vi "Thorlabs FWxC Read & Write demo.vi"() -> ()   [LabVIEW 2013]
doc: "This example shows how to acquire a power measurement using the VIs of the driver."
uses:
  <instrlib>/Thorlabs_FWxC/Thorlabs_FWxC.lvlib
panel:
  in  "Set Sensor Mode":T1(ring)
  in  "Set Speed Mode":enum16{"Slow Speed", "High Speed"}(ring)
  in  "Set Trigger Mode":enum16{"Input Mode", "Output Mode"}(ring)
  out "Get Sensor Mode":T1(ring)
  out "COM Ports":string[](array[string])
  out "Get Position":i32
  in  "Set Position":i32=5
  out "Get Speed Mode":enum16{"Slow Speed", "High Speed"}(ring)
  out "Get Trigger Mode":enum16{"Input Mode", "Output Mode"}(ring)
  out "Get Position Count":i32
  out "ID":string
  # "(c) 2020 <Thorlabs>.  ALL RIGHTS RESERVED."
  # "Connect"
  # "Set data"
  # "Read data"
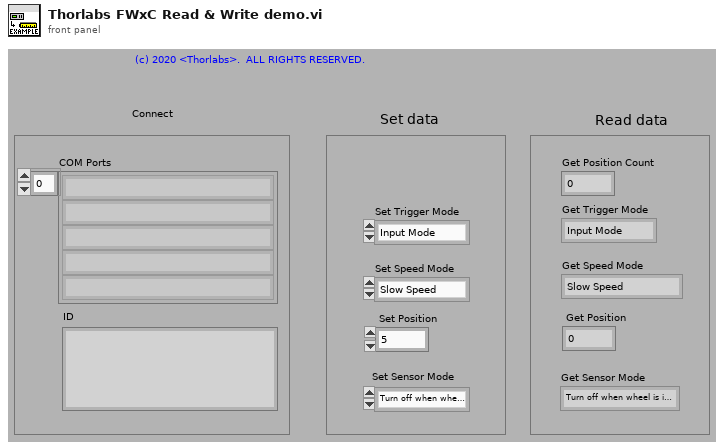
[diagram p1: front panel]
types:
  T1 = enum16{"Turn off when wheel is idle to eliminate stray light", "Remain active"}
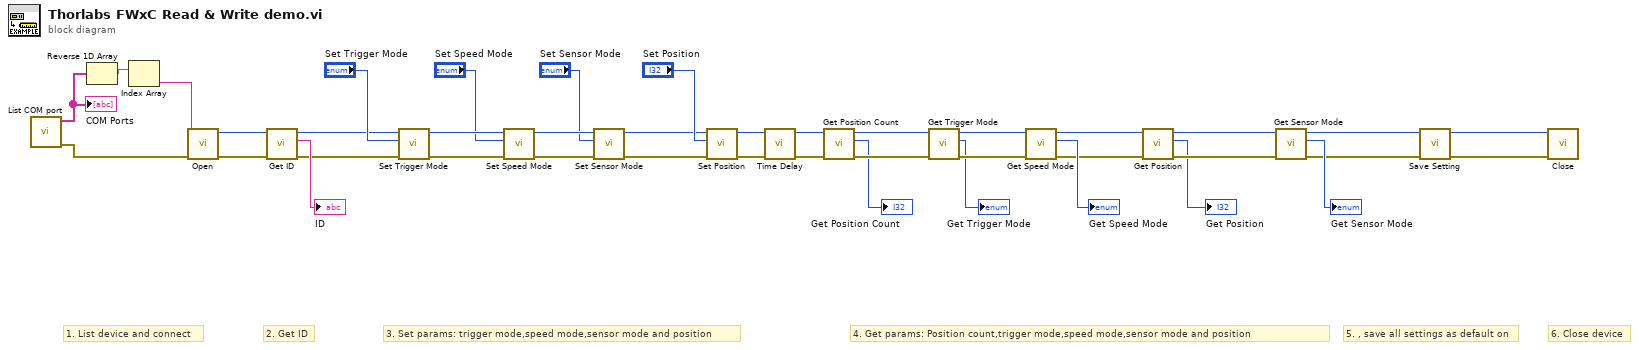
[diagram p0: block diagram]
diagram:
  # "5. , save all settings as default on"
  # "6. Close device"
  # "4. Get params: Position count,trigger mode,speed mode,sensor mode and position"
  # "3. Set params: trigger mode,speed mode,sensor mode and position"
  # "2. Get ID"
  # "1. List device and connect"
  n1 = call <instrlib>:"List COM port.vi"() -> ("error out"=w34:errorcluster, "COM Ports"=w37:string[])  [unwired: 10 in]
  "COM Ports" <- w37
  n2 = Reverse 1D Array(array=w37) -> (reversed array=w36:string[])
  n3 = Index Array(array=w36) -> (element=w35:string)  [unwired: 1 in]
  n4 = call <instrlib>:"Open.vi"("error in (no error)"=w34, "Serial Port"=w35) -> ("error out"=w38:errorcluster, "hdl out"=w39:i32)  [unwired: 7 in, 1 out]
  n5 = call <instrlib>:"Get ID.vi"("error in (no error)"=w38, "hdl in"=w39) -> ("error out"=w2:errorcluster, "ID"=→"ID":string, "hdl out"=w3:i32)  [unwired: 7 in]
  n6 = call <instrlib>:"Set Trigger Mode.vi"("error in (no error)"=w2, "Set Trigger Mode"="Set Trigger Mode", "hdl in"=w3) -> ("error out"=w13:errorcluster, "hdl out"=w19:i32)  [unwired: 7 in]
  n7 = call <instrlib>:"Set Speed Mode.vi"("error in (no error)"=w13, "Set Speed Mode"="Set Speed Mode", "hdl in"=w19) -> ("error out"=w12:errorcluster, "hdl out"=w17:i32)  [unwired: 7 in]
  n8 = call <instrlib>:"Set Sensor Mode.vi"("error in (no error)"=w12, "Set Sensor Mode"="Set Sensor Mode", "hdl in"=w17) -> ("error out"=w11:errorcluster, "hdl out"=w14:i32)  [unwired: 7 in]
  n9 = call <instrlib>:"Set Position.vi"("error in (no error)"=w11, "Set Position"="Set Position", "hdl in"=w14) -> ("error out"=w8:errorcluster, "hdl out"=w1:i32)  [unwired: 7 in]
  n10 = call "Time Delay"("error in (no error)"=w8) -> ("error out"=w7:errorcluster)  [unwired: 10 in]
  n11 = call <instrlib>:"Get Position Count.vi"("error in (no error)"=w7, "hdl in"=w1) -> ("error out"=w32:errorcluster, "Get Position Count"=→"Get Position Count":i32, "hdl out"=w33:i32)  [unwired: 7 in]
  n12 = call <instrlib>:"Get Trigger Mode.vi"("error in (no error)"=w32, "hdl in"=w33) -> ("error out"=w30:errorcluster, "Get Trigger Mode"=→"Get Trigger Mode":enum16{"Input Mode", "Output Mode"}, "hdl out"=w31:i32)  [unwired: 7 in]
  n13 = call <instrlib>:"Get Speed Mode.vi"("error in (no error)"=w30, "hdl in"=w31) -> ("error out"=w15:errorcluster, "Get Speed Mode"=→"Get Speed Mode":enum16{"Slow Speed", "High Speed"}, "hdl out"=w16:i32)  [unwired: 7 in]
  n14 = call <instrlib>:"Get Position.vi"("error in (no error)"=w15, "hdl in"=w16) -> ("error out"=w29:errorcluster, "Get Position"=→"Get Position":i32, "hdl out"=w23:i32)  [unwired: 7 in]
  n15 = call <instrlib>:"Get Sensor Mode.vi"("error in (no error)"=w29, "hdl in"=w23) -> ("error out"=w5:errorcluster, "Get Sensor Mode"=→"Get Sensor Mode":T1, "hdl out"=w22:i32)  [unwired: 7 in]
  n16 = call <instrlib>:"Save Setting.vi"("error in (no error)"=w5, "hdl in"=w22) -> ("error out"=w4:errorcluster, "hdl out"=w6:i32)  [unwired: 8 in]
  n17 = call <instrlib>:"Close.vi"("error in (no error)"=w4, "hdl in"=w6) -> ()  [unwired: 9 in, 1 out]
